vi "CSM_ExampleBrowser.vi"() -> ()   [LabVIEW 2017, in "CSM_ExampleBrowser.lvlib"]
uses:
  CSM_ExampleBrowser.lvlib
  controls/BMark_UI Data.ctl
  <vilib>/addons/analyzer/_analyzerctrls.llb/VIAnCtl Analysis App Info.ctl
  controls/BMark_Bookmark Data.ctl
  controls/BMark_VI_Identifier.ctl
  <vilib>/Utility/miscctls.llb/LVPoint32TypeDef.ctl
  _csmDoc/_Typedef/DocElement.ctl
  <vilib>/Utility/miscctls.llb/LVRowAndColumnUnsignedTypeDef.ctl
  globals/User Visible Strings.vi
  _Shared/CSM Shared.lvlib
  Communicable State Machine.lvlib
  _ui/csm-ui-support.lvlib
  _csmDoc/csmdoc.lvlib
  c14f8e0f-ff4e-477b-a84e-2a16e0658fda.vi
  _file/csm-file-support.lvlib
panel:
  in  "Localization Tool":bool
  in  "Refresh Button":bool
  in  "Zoom Factor":dbl(slide)=0.5 min=0.5 max=1.2 step=0.01 scale=0.5..1.2
  in  "ExampleTree":string(tree)
  in  "BookmarkList":i32(listbox)
  out "Preview":picture
  out "Doc":string
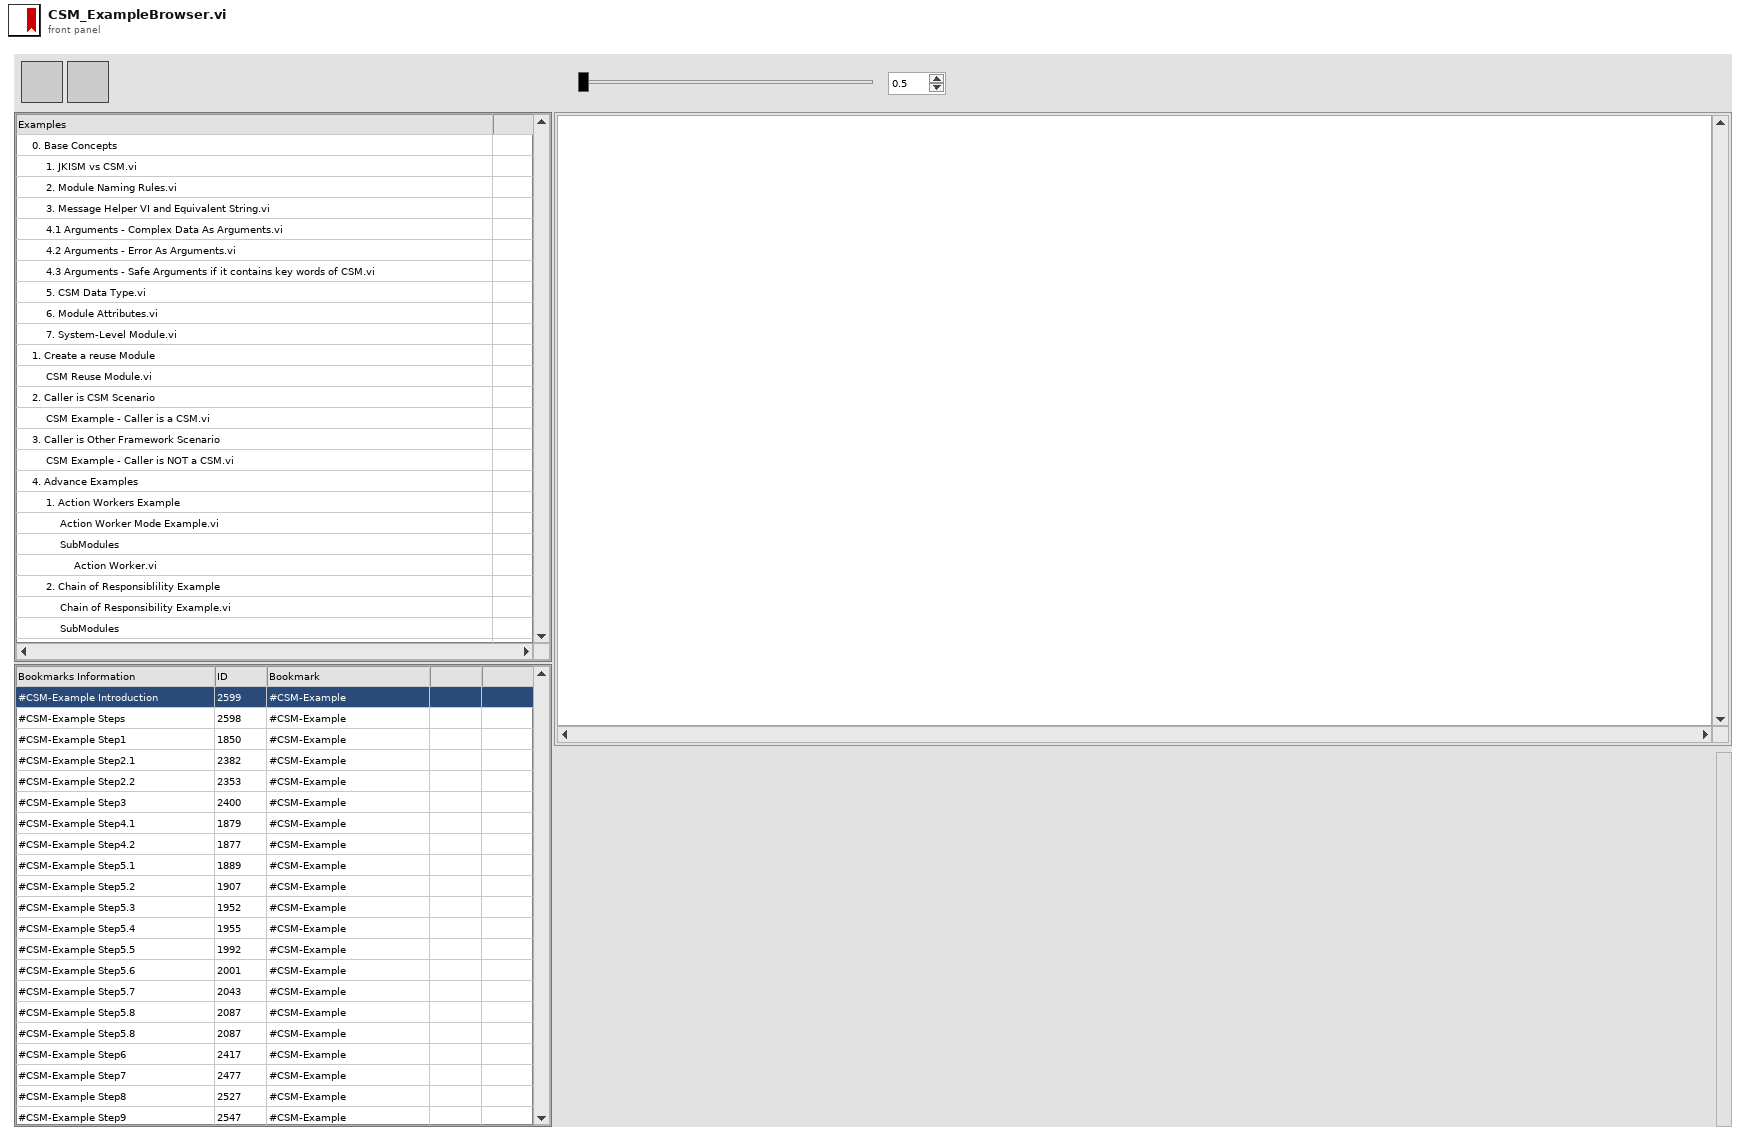
[diagram p1: front panel]
types:
  T1 = typedef "CSM_ExampleBrowser.lvlib/BMark_UI Data.ctl" = cluster{"More information":refnum<vi>, "Front Panel":refnum<vi>, "all projects":T2[], "bookmarks":T3[], "App Info":T2, "Preview image":refnum<vi>}
  T2 = typedef "VIAnCtl Analysis App Info.ctl" = cluster{"Project Name":string, "Target Name":string}
  T3 = typedef "CSM_ExampleBrowser.lvlib/BMark_Bookmark Data.ctl" = cluster{"bookmark tag":string, "full text":string, "bookmark ref":i32, "VI display name":string, "VI identifier":T4}
  T4 = typedef "CSM_ExampleBrowser.lvlib/BMark_VI_Identifier.ctl" = cluster{"Name":string, "Path":path, "App Info":T2}
  T5 = enum32{"Invalid", "Default", "Floating", "Floating/Auto-Hide", "Modal"}
  T6 = enum32{"Invalid", "Standard", "Closed", "Hidden", "Minimized", "Maximized"}
  T7 = enum32{"invalid app kind", "Development System", "Run Time System", "Student Edition", "Embedded LabVIEW", "Evaluation", "Custom"}
  T8 = enum8{"Enabled", "Disabled", "Disabled and Grayed Out"}
  T9 = typedef "csmdoc.lvlib/DocElement.ctl" = cluster{"ID":string, "Content":string[], "SubIDs":string[], "Path":string[]}
  T10 = typedef "LVRowAndColumnUnsignedTypeDef.ctl" = cluster{"Row":u32, "Column":u32}
  T11 = typedef "LVPoint32TypeDef.ctl" = cluster{"Horizontal":i32, "Vertical":i32}
  T12 = typedef "LVPointTypeDef.ctl" = cluster{"Horizontal":i16, "Vertical":i16}
  T13 = cluster{"Core":cluster{"Current VI Reference":refnum<vi>, "Close Panel on Exit?":bool}, "root":path, "ExampleMarkdowns":path[], "PreviewMouseDown":bool, "PreviewMouseDownCoords":T11, "PreviewMouseDownOrigin":T11, "DocMap":variant, "tempfile":path}
  T14 = typedef "LVRectTypeDef.ctl" = cluster{"Left":i16, "Top":i16, "Right":i16, "Bottom":i16}
  T15 = cluster{"Current VI Reference":refnum<vi>, "Close Panel on Exit?":bool}
  T16 = cluster{"Core":cluster{"Current VI Reference":refnum<vi>, "Close Panel on Exit?":bool}, "root":path, "PreviewMouseDown":bool, "PreviewMouseDownCoords":T11, "PreviewMouseDownOrigin":T11}
  T17 = typedef "csmdoc.lvlib/DocNote.ctl" = cluster{"ID":string, "Content":string, "Type":string}
  T18 = typedef "LVBookmarkInfoTypeDef.ctl" = cluster{"Bookmark Reference":u32, "Bookmark Tag":string, "Label Text":string}[]
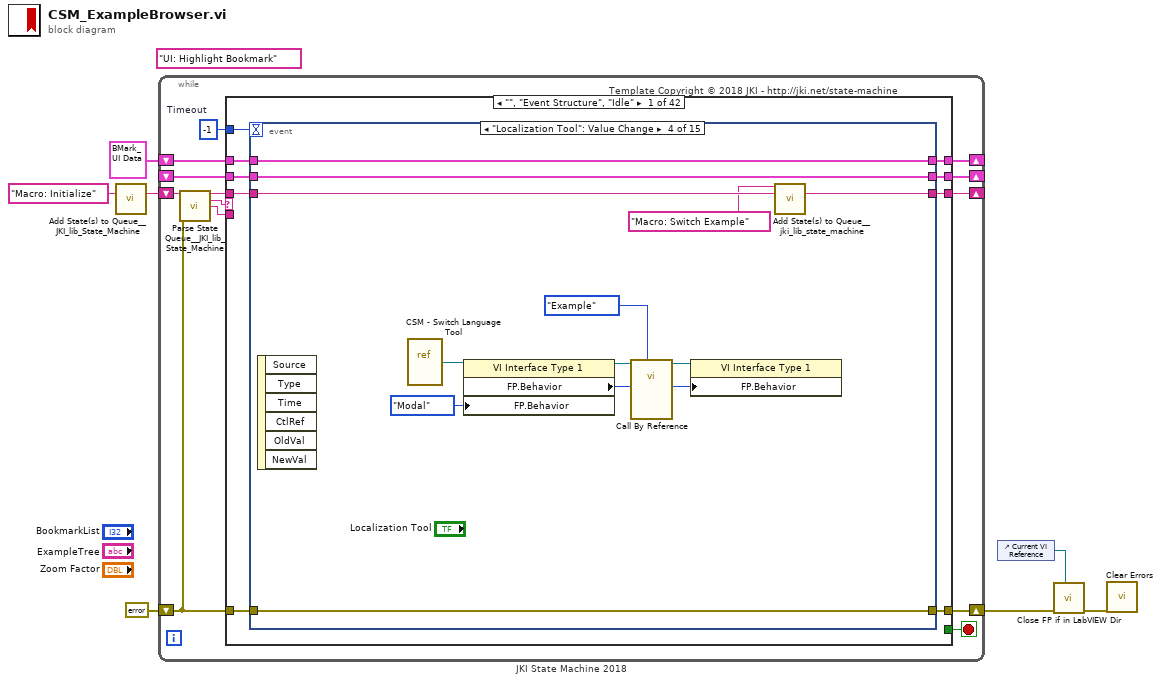
[diagram p0: block diagram]
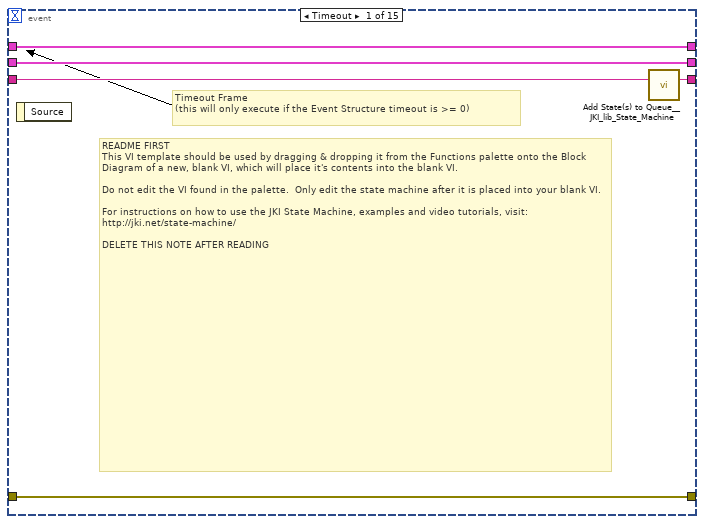
[diagram p2: hidden frame]
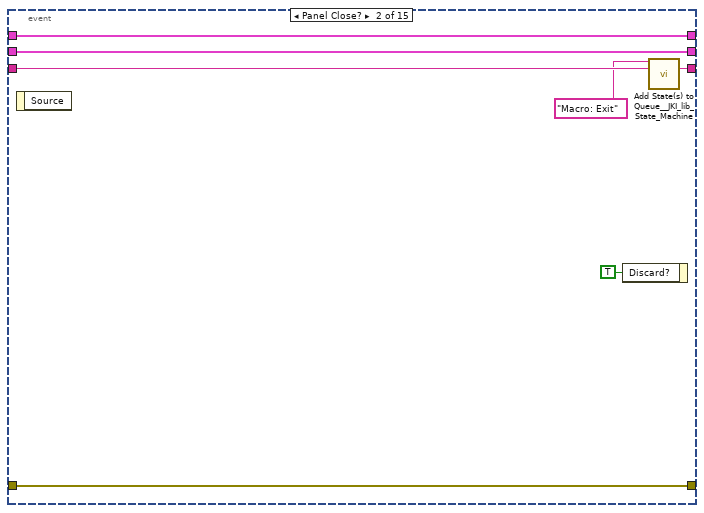
[diagram p3: hidden frame]
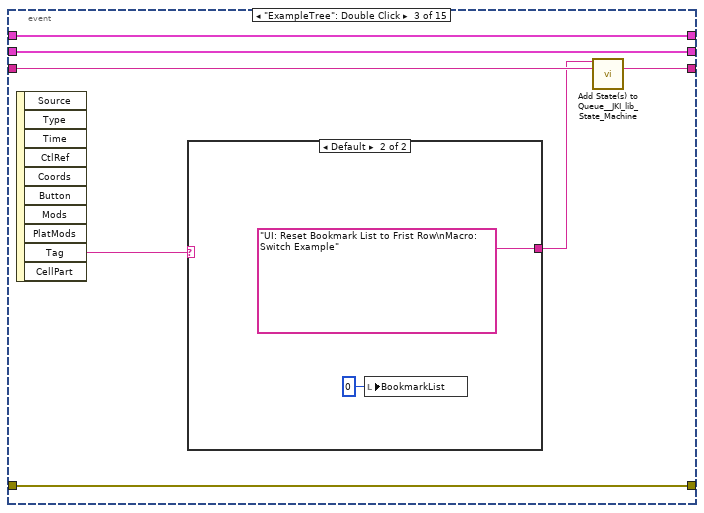
[diagram p4: hidden frame]
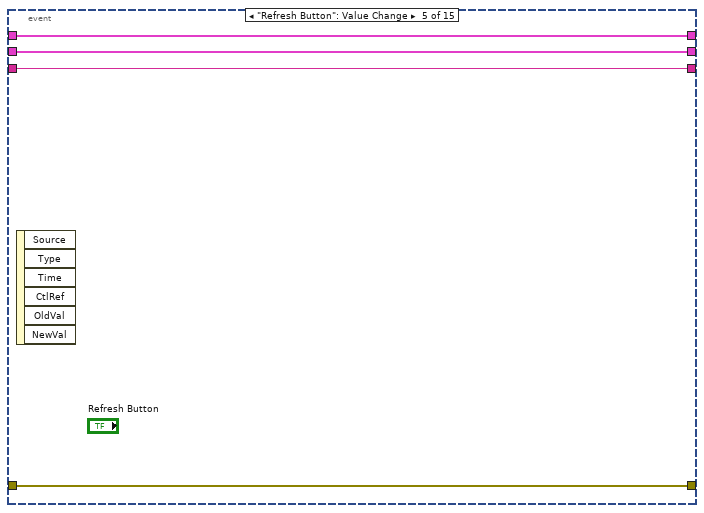
[diagram p6: hidden frame]
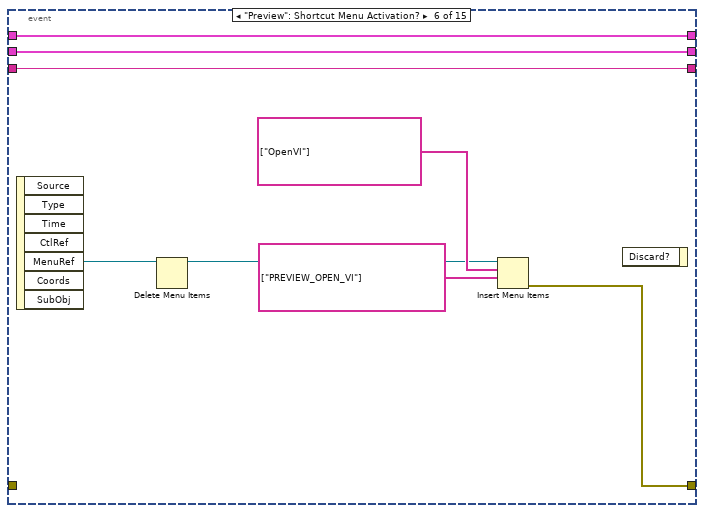
[diagram p7: hidden frame]
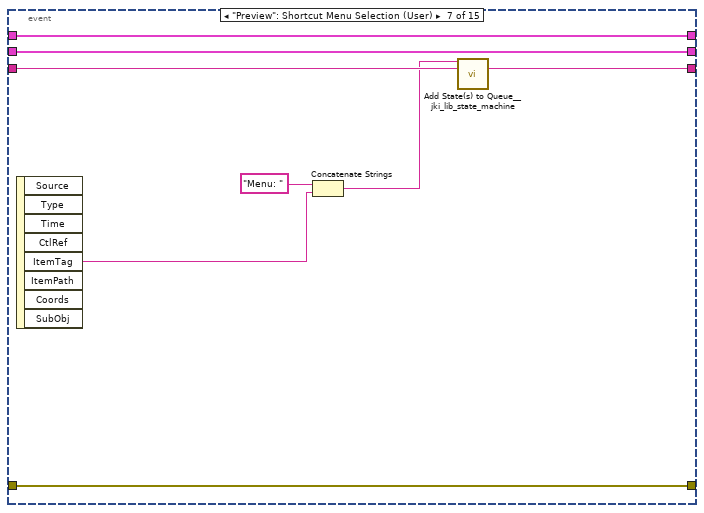
[diagram p8: hidden frame]
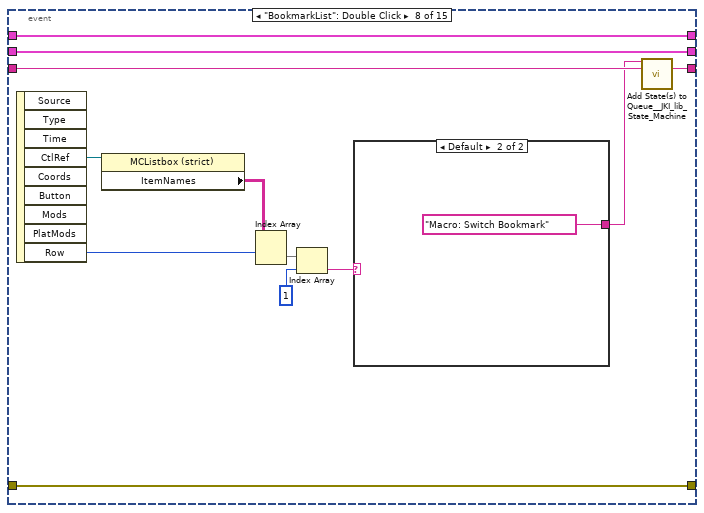
[diagram p9: hidden frame]
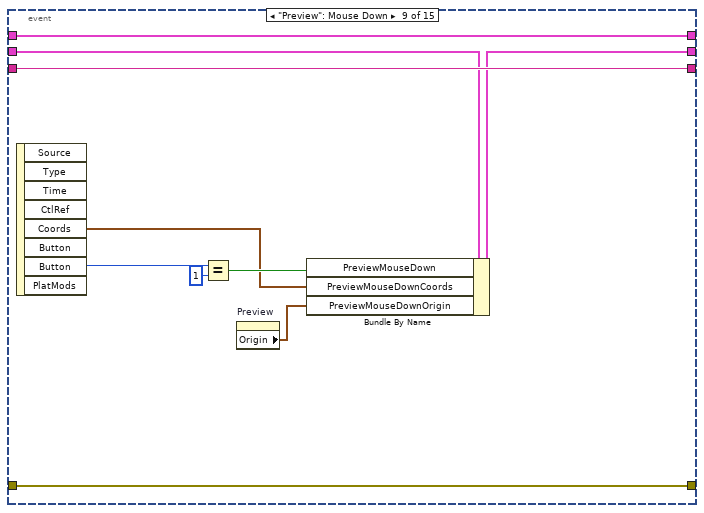
[diagram p11: hidden frame]
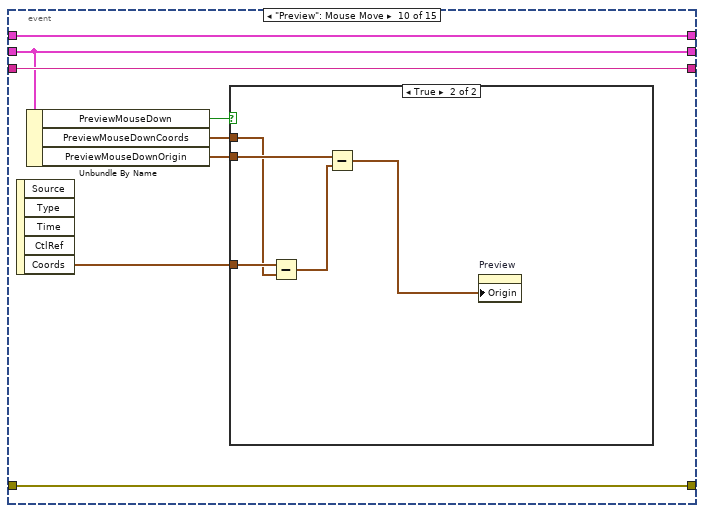
[diagram p12: hidden frame]
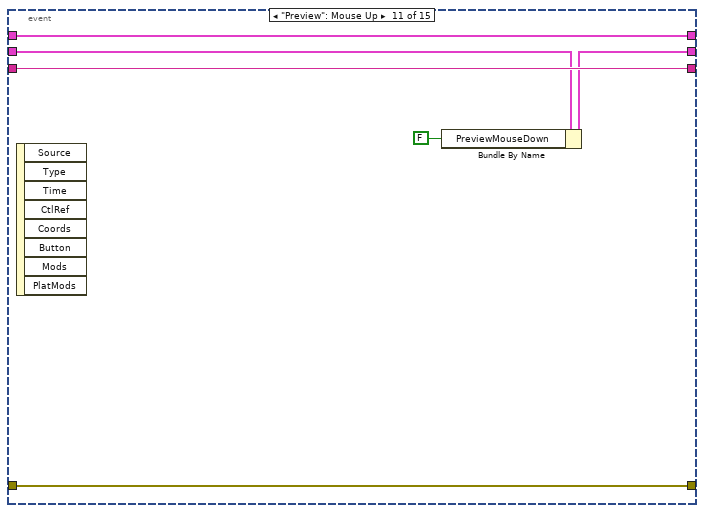
[diagram p14: hidden frame]
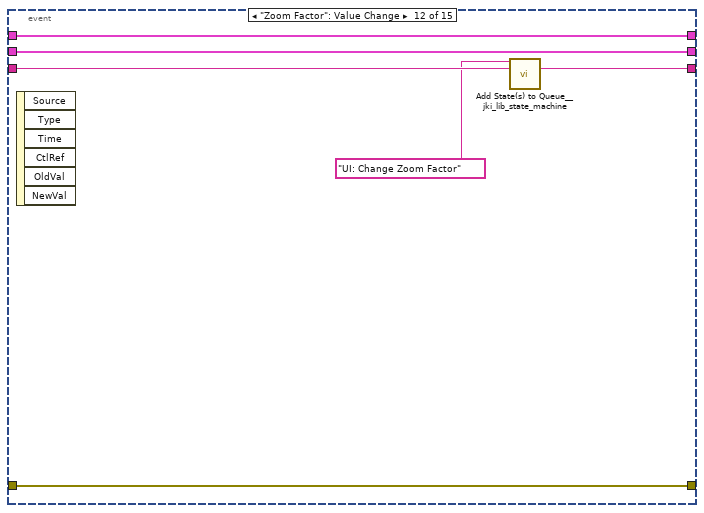
[diagram p15: hidden frame]
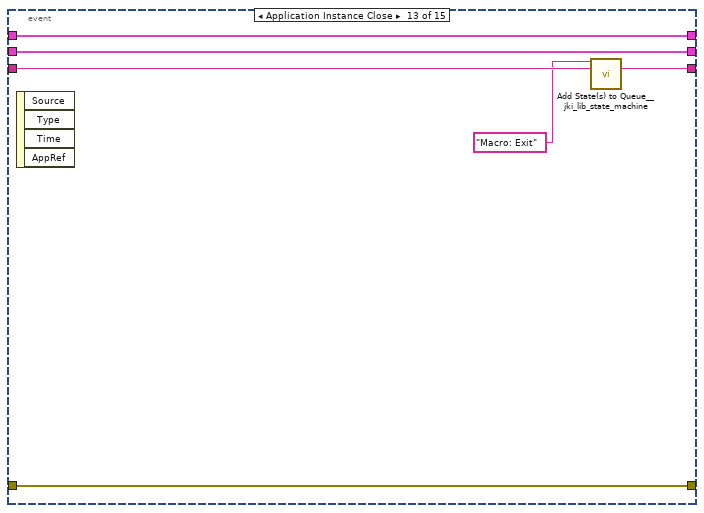
[diagram p16: hidden frame]
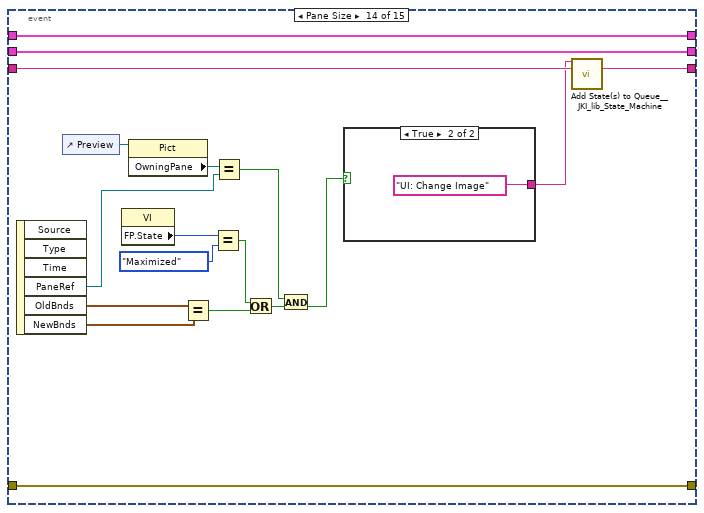
[diagram p17: hidden frame]
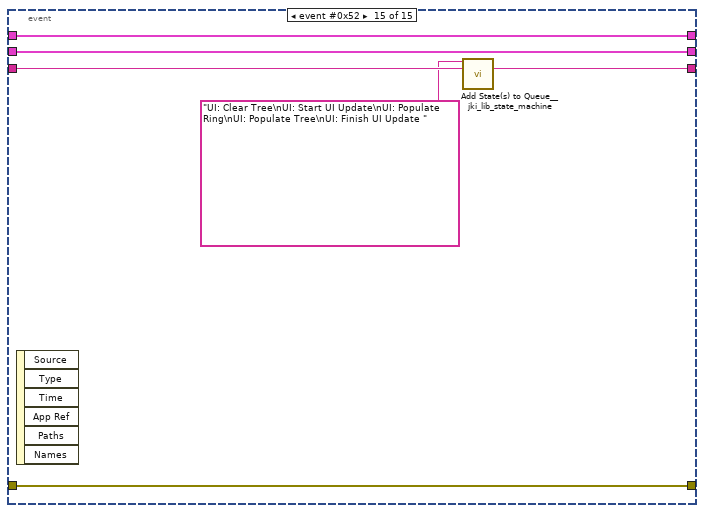
[diagram p19: hidden frame]
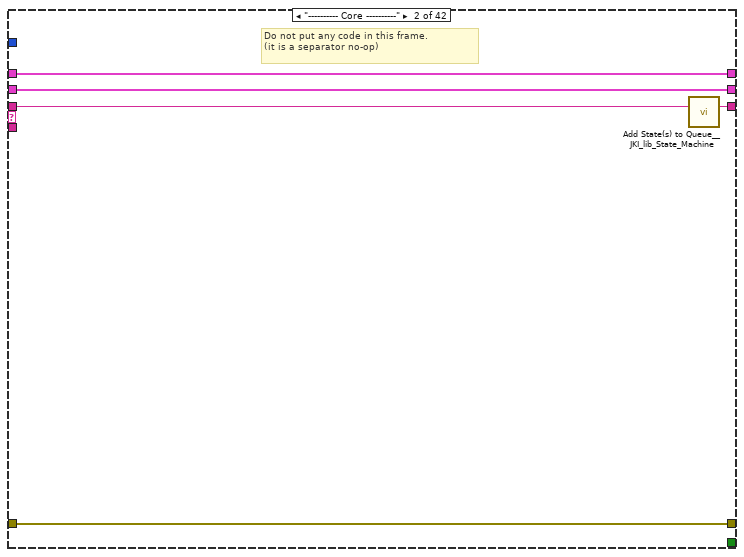
[diagram p20: hidden frame]
diagram:
  (unwired) "UI: Highlight Bookmark" ("Message")
  n1 = call <vilib>:"Add State(s) to Queue__JKI_lib_State_Machine.vi"("State(s) in (\"\")"="Macro: Initialize") -> ("States Out"=w6:string)  [unwired: 14 in]
  n2 = while "JKI State Machine 2018" {
    shift-right: [w13] -> _
    shift-left: _ -> [w12]
    shift-right: [w16] -> w1
    shift-left: errorcluster {"status"=FALSE, "code"=0, "source"=""} ("error out") -> [w10]
    shift-right: [w15] -> _
    shift-left: w6 -> [w17]
    shift-right: [w9] -> _
    shift-left: T1 {"More information"=refnum, "Front Panel"=refnum, "all projects"=[], "bookmarks"=[], "App Info"={"Project Name"="", "Target Name"=""}, "Preview image"=refnum} ("Data Cluster") -> [w8]
    stop <- w14 stop-if-true
    w11 = -1  # Timeout
    # "Template Copyright © 2018 JKI - http://jki.net/state-machine"
    n3 = call <vilib>:"Parse State Queue__JKI_lib_State_Machine.vi"("State Queue"=w17, "Error In (no error)"=w10) -> ("Remaining States"=w19:string, "Current State"=w20:string, "Arguments"=w18:string)  [unwired: 11 in]
    n4 = case shown="\"\", \"Event Structure\", \"Idle\"" w20 {
      selector: w20 -> [_ _ w168 _ _ _ _ _ _ _ _ _ _ _ _ _ _ _ _ _ _ _ _ _ _ _ _ _ _ _ _ _ _ _ _ _ _ _ _ _ _ _]
      tunnel: w19 -> [w29 w166 w172 w192 w199 w205 w210 w227 w244 w260 w274 w285 w290 w300 w302 w317 w320 w329 w338 w341 w354 w360 w376 w425 w432 w434 w452 w477 w489 w560 w568 w571 w584 w590 w596 w602 w613 w618 w626 w631 w662 w681]
      tunnel: w18 -> [_ _ _ _ _ _ _ _ _ _ _ _ _ _ _ _ _ _ _ _ _ _ w363 _ w430 _ _ w472 w483 w556 _ _ _ _ _ _ _ _ _ _ _ _]
      tunnel: w12 -> [w27 w163 w170 w185 w196 w203 w207 w211 _ w259 w272 w280 w287 w298 w306 w316 w323 w328 w337 w340 w346 w359 w375 w424 w431 w437 w448 w475 w485 w559 w567 w575 w581 w587 w593 w599 w610 w615 w620 w629 w657 w675]
      tunnel: [w26 w164 w174 w189 errorcluster {"status"=FALSE, "code"=0, "source"=""} ("error out") w202 w208 w224 w241 w261 w275 w281 w288 w297 w305 w318 w324 w330 w336 _ w345 w361 w366 _ _ _ _ w473 w486 w561 w569 w579 w582 w588 w594 w600 w611 w616 w627 _ w653 w679] -> w16
      tunnel: w10 -> [w25 w164 w173 w189 w195 w202 w208 w224 w241 w261 w275 w282 w288 w297 _ w318 w324 w330 _ _ _ w361 _ _ _ _ _ w474 w487 w561 w569 w579 w582 w588 w594 w600 w611 w616 w627 _ _ w679]
      tunnel: [w28 w165 w171 w191 w198 w204 w209 w226 w243 w260 w274 w284 w289 w299 w303 w317 w321 w329 w338 w341 w354 w360 w376 w425 w432 w435 w452 w476 w488 w560 w568 w572 w583 w589 w595 w601 w612 w617 w626 w631 w661 w680] -> w15
      tunnel: [_ _ _ _ _ TRUE _ _ _ _ _ _ _ _ _ _ _ _ _ _ _ _ _ _ _ _ _ _ _ _ _ _ _ _ _ _ _ _ _ _ _ _] -> w14
      tunnel: [w24 w163 w170 w190 w196 w203 w207 w211 w237 w257 w269 w280 w287 w298 w306 w316 w323 w328 w337 w340 w346 w359 w375 w424 w431 w437 w450 w475 w485 w559 w567 w575 w581 w587 w593 w599 w610 w615 w620 w628 w655 w675] -> w13
      tunnel: w11 -> [w23 _ _ _ _ _ _ _ _ _ _ _ _ _ _ _ _ _ _ _ _ _ _ _ _ _ _ _ _ _ _ _ _ _ _ _ _ _ _ _ _ _]
      tunnel: [w22 w162 w167 w179 w193 w200 w206 w215 w231 w258 w273 w279 w286 w296 w304 w308 w322 w325 w333 w339 w348 w356 w367 w423 w429 w447 w451 w471 w482 w558 w566 w578 w580 w585 w591 w597 w603 w614 w625 w630 w660 w678] -> w9
      tunnel: w8 -> [w21 w162 w167 w179 w193 w200 w206 w216 w231 w258 w273 w279 w286 w296 w304 w308 w322 w325 w332 w339 w348 w356 w367 w423 w429 w447 w451 w471 w482 w558 w566 w578 w580 w585 w591 w597 w603 w614 w625 w630 w660 w678]
      frame "", "Event Structure", "Idle" {
        n5 = event shown="[3] \"Localization Tool\": Value Change" {
          selector: _ -> [_ _ _ _ _ _ _ _ _ _ _ _ _ _ _]
          dyn-events: _ -> [_ _ _ _ _ _ _ _ _ _ _ _ _ _ _]
          timeout: w23 -> [_ _ _ _ _ _ _ _ _ _ _ _ _ _ _]
          tunnel: w29 -> [w34 w41 w44 w52 w66 w74 w78 w90 w105 w113 w124 w126 w132 w144 w157]
          tunnel: [w33 w40 w45 w53 w66 w74 w79 w91 w105 w113 w124 w127 w133 w145 w158] -> w28
          tunnel: w27 -> [w31 w38 w47 w61 w64 w73 w81 w93 w103 w110 w122 w129 w135 w153 w160]
          tunnel: [w32 w39 w48 w62 w65 w68 w82 w94 w104 w112 w123 w130 w136 w154 w161] -> w26
          tunnel: w25 -> [w32 w39 w48 w62 w65 _ w82 w94 w104 w112 w123 w130 w136 w154 w161]
          tunnel: [w31 w38 w47 w61 w64 w73 w81 w93 w101 w110 w120 w129 w135 w153 w160] -> w24
          tunnel: [w30 w35 w46 w60 w63 w72 w80 w92 w102 w111 w121 w128 w134 w152 w159] -> w22
          tunnel: w21 -> [w30 w35 w46 w60 w63 w72 w80 w92 w102 w111 w121 w128 w134 w152 w159]
          event Timeout {
            # "README FIRST\nThis VI template should be used by dragging & dropping it from the Functions palette onto the Block Diagram of a new, blank VI, which will place it's contents into the blank VI.\n\nDo not edit the VI found in the palette.  Only edit the state machine after it is placed into your blank VI.\n\nFor instructions on how to use the JKI State Machine, examples and video tutorials, visit:\nhttp://jki.net/state-machine/\n\nDELETE THIS NOTE AFTER READING"
            # "Timeout Frame\n(this will only execute if the Event Structure timeout is >= 0)"
            n6 = event-data() -> ()  [unwired: 1 in, 1 out]
            n7 = call <vilib>:"Add State(s) to Queue__JKI_lib_State_Machine.vi"("State(s) in (\"\")"=w34) -> ("States Out"=w33:string)  [unwired: 14 in]
          }
          event Panel Close? {
            n8 = event-data() -> ()  [unwired: 1 in, 1 out]
            n9 = event-data("Discard?"=TRUE) -> ()  [unwired: 1 in, 1 out]
            n10 = call <vilib>:"Add State(s) to Queue__JKI_lib_State_Machine.vi"("State(s) in Front (\"\")"="Macro: Exit", "State(s) in (\"\")"=w41) -> ("States Out"=w40:string)  [unwired: 13 in]
          }
          event "ExampleTree": Double Click {
            n11 = event-data() -> ("Tag"=w42:string)  [unwired: 1 in, 9 out]
            n12 = case shown="Default" w42 {
              tunnel: [_ "UI: Reset Bookmark List to Frist Row\nMacro: Switch Example" ("Message")] -> w43
              frame "" {
              }
              frame Default {
                n13 = local write "BookmarkList"(0 ("BookmarkList")) -> ()
              }
            }
            n14 = call <vilib>:"Add State(s) to Queue__JKI_lib_State_Machine.vi"("State(s) in Front (\"\")"=w43, "State(s) in (\"\")"=w44) -> ("States Out"=w45:string)  [unwired: 13 in]
          }
          event "Localization Tool": Value Change {
            n15 = event-data() -> ()  [unwired: 1 in, 6 out]
            n16 = vi-ref "CSM - Switch Language Tool.vi"() -> (w59:refnum<vi>)
            n17 = property class="VI Interface Type 1"(reference=w59, "FP.Behavior"=T5."Modal" ("Front Panel Window:Behavior")) -> (reference out=w56:refnum<vi>, "FP.Behavior"=w57:T5)  [unwired: 1 in, 1 out]
            n18 = call-by-ref "?"(reference=w56, "Type"=enum16{"VI Description", "Example"}."Example") -> (reference out=w55:refnum<vi>)  [unwired: 12 in, 1 out]
            n19 = property class="VI Interface Type 1"(reference=w55, "FP.Behavior"=w57) -> ()  [unwired: 1 in, 2 out]
            n20 = call <vilib>:"Add State(s) to Queue__jki_lib_state_machine.vi"("State(s) in Front (\"\")"="Macro: Switch Example" ("State(s) in Front (\"\")"), "State(s) in (\"\")"=w52) -> ("States Out"=w53:string)  [unwired: 13 in]
          }
          event "Refresh Button": Value Change {
            n21 = event-data() -> ()  [unwired: 1 in, 6 out]
          }
          event "Preview": Shortcut Menu Activation? {
            n22 = event-data() -> ("MenuRef"=w71:refnum<k9>)  [unwired: 1 in, 6 out]
            n23 = Delete Menu Items(9:w71) -> (3:w67:refnum<k9>)  [unwired: 3 in, 1 out]
            n24 = Insert Menu Items(7:string[] ["PREVIEW_OPEN_VI"] ("item names"), 8:string[] ["OpenVI"] ("item names"), 9:w67) -> (0:w68:errorcluster)  [unwired: 3 in, 2 out]
            n25 = event-data() -> ()  [unwired: 2 in, 1 out]
          }
          event "Preview": Shortcut Menu Selection (User) {
            n26 = event-data() -> ("ItemTag"=w76:string)  [unwired: 1 in, 7 out]
            n27 = Concatenate Strings("Menu: ", w76) -> (w75:string)
            n28 = call <vilib>:"Add State(s) to Queue__jki_lib_state_machine.vi"("State(s) in Front (\"\")"=w75, "State(s) in (\"\")"=w78) -> ("States Out"=w79:string)  [unwired: 13 in]
          }
          event "BookmarkList": Double Click {
            n29 = event-data() -> ("CtlRef"=w88:refnum<vi>, "Row"=w86:i32)  [unwired: 1 in, 7 out]
            n30 = property class="MCListbox (strict)"(reference=w88) -> ("ItemNames"=w87:string[][])  [unwired: 1 in, 2 out]
            n31 = Index Array(array=w87, index (row)=w86) -> (element=w85:string[])  [unwired: 1 in]
            n32 = Index Array(array=w85, index=1) -> (element=w84:string)
            n33 = case shown="Default" w84 {
              tunnel: [_ "Macro: Switch Bookmark" ("Message")] -> w89
              frame "" {
              }
              frame Default {
              }
            }
            n34 = call <vilib>:"Add State(s) to Queue__JKI_lib_State_Machine.vi"("State(s) in Front (\"\")"=w89, "State(s) in (\"\")"=w90) -> ("States Out"=w91:string)  [unwired: 13 in]
          }
          event "Preview": Mouse Down {
            n35 = event-data() -> ("Coords"=w97:T11, "Button"=w100:u16)  [unwired: 1 in, 6 out]
            n36 = Equal?(x=w100, y=u16 1) -> (x = y?=w99:bool)
            n37 = property on="Preview" class="Pict"() -> ("Origin"=w96:T12)  [unwired: 2 in, 2 out]
            n38 = Bundle By Name(cluster=w103, "PreviewMouseDown"=w99, "PreviewMouseDownCoords"=w97, "PreviewMouseDownOrigin"=w96) -> (w101:T13)
          }
          event "Preview": Mouse Move {
            n39 = event-data() -> ("Coords"=w107:T11)  [unwired: 1 in, 4 out]
            n40 = Unbundle By Name(w110) -> ("PreviewMouseDown"=w109:bool, "PreviewMouseDownCoords"=w108:T11, "PreviewMouseDownOrigin"=w106:T11)
            n41 = case shown="True" w109 {
              tunnel: w108 -> [_ w116]
              tunnel: w107 -> [_ w117]
              tunnel: w106 -> [_ w118]
              frame False {
              }
              frame True {
                n42 = Subtract(x=w117, y=w116) -> (x-y=w115:T11)
                n43 = Subtract(x=w118, y=w115) -> (x-y=w114:T11)
                n44 = property on="Preview" class="Pict"("Origin"=w114) -> ()  [unwired: 2 in, 2 out]
              }
            }
          }
          event "Preview": Mouse Up {
            n45 = event-data() -> ()  [unwired: 1 in, 8 out]
            n46 = Bundle By Name(cluster=w122, "PreviewMouseDown"=FALSE) -> (w120:T13)
          }
          event "Zoom Factor": Value Change {
            n47 = event-data() -> ()  [unwired: 1 in, 6 out]
            n48 = call <vilib>:"Add State(s) to Queue__jki_lib_state_machine.vi"("State(s) in Front (\"\")"="UI: Change Zoom Factor" ("State(s) in Front (\"\")"), "State(s) in (\"\")"=w126) -> ("States Out"=w127:string)  [unwired: 13 in]
          }
          event Application Instance Close {
            n49 = event-data() -> ()  [unwired: 1 in, 4 out]
            n50 = call <vilib>:"Add State(s) to Queue__jki_lib_state_machine.vi"("State(s) in Front (\"\")"="Macro: Exit" ("State(s) in Front (\"\")"), "State(s) in (\"\")"=w132) -> ("States Out"=w133:string)  [unwired: 13 in]
          }
          event Pane Size {
            n51 = event-data() -> ("PaneRef"=w139:refnum<vi>, "OldBnds"=w147:T14, "NewBnds"=w146:T14)  [unwired: 1 in, 3 out]
            n52 = control-ref of="Preview"() -> (w141:refnum<vi>)
            n53 = property class="VI"() -> ("FP.State"=w151:T6)  [unwired: 2 in, 2 out]
            n54 = property class="Pict"(reference=w141) -> ("OwningPane"=w140:refnum<vi>)  [unwired: 1 in, 2 out]
            n55 = Equal?(x=w147, y=w146) -> (x = y?=w148:bool)
            n56 = Equal?(x=w151, y=T6."Maximized" ("Front Panel Window:State")) -> (x = y?=w149:bool)
            n57 = Equal?(x=w140, y=w139) -> (x = y?=w137:bool)
            n58 = Or(x=w149, y=w148) -> (x .or. y?=w142:bool)
            n59 = And(x=w137, y=w142) -> (x .and. y?=w138:bool)
            n60 = case shown="True" w138 {
              tunnel: [_ "UI: Change Image" ("Message")] -> w143
              frame False {
              }
              frame True {
              }
            }
            n61 = call <vilib>:"Add State(s) to Queue__JKI_lib_State_Machine.vi"("State(s) in Front (\"\")"=w143, "State(s) in (\"\")"=w144) -> ("States Out"=w145:string)  [unwired: 13 in]
          }
          event event #0x52 {
            n62 = event-data() -> ()  [unwired: 1 in, 6 out]
            n63 = call <vilib>:"Add State(s) to Queue__jki_lib_state_machine.vi"("State(s) in Front (\"\")"="UI: Clear Tree\nUI: Start UI Update\nUI: Populate Ring\nUI: Populate Tree\nUI: Finish UI Update " ("State(s) in Front (\"\")"), "State(s) in (\"\")"=w157) -> ("States Out"=w158:string)  [unwired: 13 in]
          }
        }
      }
      frame "---------- Core ----------" {
        # "Do not put any code in this frame.\n(it is a separator no-op)"
        n64 = call <vilib>:"Add State(s) to Queue__JKI_lib_State_Machine.vi"("State(s) in (\"\")"=w166) -> ("States Out"=w165:string)  [unwired: 14 in]
      }
      frame Default {
        w177 = 42 items=["No error", "Argument error", "Memory is full", "Out of zone", "End of file", "File already open", "Generic file I/O error", "File not found", "File permission error", "Disk is full", "Duplicate path", "Too many files open", "System feature not enabled", "Resource file not found", "Cannot add resource", "Resource not found", "Image not found", "Image memory error", "Pen does not exist", "Config type invalid", "Config token not found", "Config parse error", "Config memory error", "Bad external code format", "Bad external code offset", "External code not present", "Null window", "Destroy window error", "Null menu", "Print aborted", "Bad print record", "Print driver error", "Windows error during printing", "Memory error during printing", "Print dialog error", "Generic print error", "Invalid device refnum", "Device not found", "Device parameter error", "Device unit error", "Cannot open device", "Device call aborted", "Generic error", "Cancelled by user", "Object ID too low", "Object ID too high", "Object not in heap", "Unknown heap", "Unknown object (invalid DefProc)", "Unknown object (DefProc not in table)", "Message out of range", "Invalid (null) method", "Unknown message", "Manager call not supported", "Bad address", "Network operation in progress", "Network operation timed out", "Connection is busy", "Network attribute not supported", "Network error", "Address in use", "System out of memory", "Connection aborted", "Connection refused", "Not connected", "Already connected", "Connection closed", "Initialization error (interapplication manager)", "Bad occurrence", "Wait on unbound occurrence handler", "Occurrence queue overflow", "Datalog type conflict", "Unused", "Unrecognized type (interapplication manager)", "Memory corrupt", "Failed to make temporary DLL", "Old CIN version", "Drag socket not found", "Failed to load drop-object", "Failed to register OLE object", "Failed to release OLE object", "Format specifier type mismatch", "Unknown format specifier", "Too few format specifiers", "Too many format specifiers", "Scan failed", "Newer CIN version", "Error converting to variant", "Runtime menu error", "Password tampered", "Variant attribute not found", "Incompatible variant data type", "Event data is not available", "Event Store is not present", "Occurrence is not found", "Event Queue is not created", "Event info is not available", "Refnum passed is NULL", "Error retrieving Class GUID", "Error retrieving CoClass GUID", "Error retrieving TypeLib GUID.", "Bad built application magic bytes.", "Specific driver is different from the specific driver associated with the Logical Name.", "There is no session opened to the class driver.", "Max Error", "MAX - Error with config objects", "MAX - Error loading configuration", "MAX - Group not supported"]
        # "Current State"
        # "Do not delete, rename, or modify this frame.\n(this is used to capture unhandled states and typos)"
        # "Handle mistyped state name (developer tool)"
        n65 = Format Into String(format string="Software Exception: Unhandled State \"%s\"." ("message"), error in=w173, w168) -> (resulting string=w176:string, error out=w175:errorcluster)  [unwired: 1 in]
        n66 = call <vilib>:"Error Cluster From Error Code.vi"("show call chain? (False)"=TRUE, "error in (no error)"=w175, "error message (\"\")"=w176, "error code (0)"=w177) -> ("error out"=w174:errorcluster)  [unwired: 5 in]
        n67 = call <vilib>:"Add State(s) to Queue__JKI_lib_State_Machine.vi"("State(s) in (\"\")"=w172) -> ("States Out"=w171:string)  [unwired: 14 in]
      }
      frame "Initialize Core Data" {
        # "Do not delete, rename, or modify this frame.\n(this is used to determine panel behavior on exit)"
        # "originally closed?"
        # "exe?"
        # "If panel starts closed or is an EXE, then close it when we exit"
        n68 = property class="VI"() -> ("FP.State"=w182:T6)  [unwired: 2 in, 2 out]
        n69 = property class="App"() -> ("App.Kind"=w188:T7)  [unwired: 2 in, 2 out]
        n70 = control-ref of="Current VI Reference"() -> (w183:refnum<vi>)
        n71 = Equal?(x=w182, y=T6."Closed" ("Front Panel Window:State")) -> (x = y?=w180:bool)
        n72 = Equal?(x=w188, y=T7."Run Time System" ("Application:Kind")) -> (x = y?=w186:bool)
        n73 = Or(x=w180, y=w186) -> (x .or. y?=w184:bool)
        n74 = Bundle By Name(cluster=w185, "Core.Current VI Reference"=w183, "Core.Close Panel on Exit?"=w184) -> (w190:T13)
        n75 = call <vilib>:"Add State(s) to Queue__JKI_lib_State_Machine.vi"("State(s) in (\"\")"=w192) -> ("States Out"=w191:string)  [unwired: 14 in]
      }
      frame "Error Handler" {
        # "Unhandled Error -- Display it"
        # "Handle any errors here.\nYou can also output any states to clean-up after errors occur"
        # "Clear error"
        n76 = call <vilib>:"General Error Handler.vi"("error in (no error)"=w195) -> ()  [unwired: 10 in, 5 out]
        n77 = call <vilib>:"Add State(s) to Queue__JKI_lib_State_Machine.vi"("State(s) in Front (\"\")"="/* Post Error States", "State(s) in (\"\")"=w199) -> ("States Out"=w198:string)  [unwired: 13 in]
      }
      frame "Exit" {
        # "Do not put any code in this frame.\n(No errors that occur here will be handled.)"
        n78 = call <vilib>:"Add State(s) to Queue__JKI_lib_State_Machine.vi"("State(s) in (\"\")"=w205) -> ("States Out"=w204:string)  [unwired: 14 in]
      }
      frame "---------- Data ----------" {
        # "Do not put any code in this frame.\n(It is a separator no-op. You can make a copy of this frame to create a new Data frame)"
        n79 = call <vilib>:"Add State(s) to Queue__JKI_lib_State_Machine.vi"("State(s) in (\"\")"=w210) -> ("States Out"=w209:string)  [unwired: 14 in]
      }
      frame "Data: Initialize Refs" {
        w212 = T11 {"Horizontal"=0, "Vertical"=0}  # PreviewMouseDownOrigin
        w213 = T11 {"Horizontal"=0, "Vertical"=0}  # PreviewMouseDownCoords
        w214 = FALSE  # PreviewMouseDown
        w223 = T15 {"Current VI Reference"=refnum, "Close Panel on Exit?"=FALSE}  # Core
        w219 = path ""  # root
        # "Initialize the shift-register data, here.\n(data names are defined by what you wire into the bundle function)"
        n80 = property class="VI"() -> ("Panel"=w217:refnum<vi>)  [unwired: 2 in, 2 out]
        n81 = control-ref of="Preview"() -> (w218:refnum<vi>)
        n82 = Bundle By Name(cluster=w216, "Front Panel"=w217, "Preview image"=w218) -> (w215:T1)
        n83 = Bundle("Core"=w223, "root"=w219, "PreviewMouseDown"=w214, "PreviewMouseDownCoords"=w213, "PreviewMouseDownOrigin"=w212) -> (w225:T16)  [unwired: 1 in]
        n84 = call "CSM - user.lib Dir.vi"() -> ("<LabVIEW>"=w222:path)  [unwired: 2 in, 1 out]
        n85 = Build Path(base path=w222, name or relative path="Example") -> (appended path=w220:path)
        n86 = Bundle By Name(cluster=w225, "root"=w220) -> ()  [unwired: 1 out]
        n87 = call <vilib>:"Add State(s) to Queue__JKI_lib_State_Machine.vi"("State(s) in (\"\")"=w227) -> ("States Out"=w226:string)  [unwired: 14 in]
      }
      frame "Data: Initialize" {
        w228 = path ""  # tempfile
        w229 = variant  # DocMap
        w230 = path[] []  # ExampleMarkdowns
        w232 = T11 {"Horizontal"=0, "Vertical"=0}  # PreviewMouseDownOrigin
        w233 = T11 {"Horizontal"=0, "Vertical"=0}  # PreviewMouseDownCoords
        w234 = FALSE  # PreviewMouseDown
        w240 = T15 {"Current VI Reference"=refnum, "Close Panel on Exit?"=FALSE}  # Core
        w235 = path ""  # root
        n88 = Bundle("Core"=w240, "root"=w235, "ExampleMarkdowns"=w230, "PreviewMouseDown"=w234, "PreviewMouseDownCoords"=w233, "PreviewMouseDownOrigin"=w232, "DocMap"=w229, "tempfile"=w228) -> (w242:T13)  [unwired: 1 in]
        n89 = call "CSM - user.lib Dir.vi"() -> ("<LabVIEW>"=w239:path)  [unwired: 2 in, 1 out]
        n90 = Build Path(base path=w239, name or relative path="examples\\NEVSTOP\\Communicable State Machine(CSM)") -> (appended path=w236:path)
        n91 = Bundle By Name(cluster=w242, "root"=w236) -> (w237:T13)
        n92 = call <vilib>:"Add State(s) to Queue__JKI_lib_State_Machine.vi"("State(s) in (\"\")"=w244) -> ("States Out"=w243:string)  [unwired: 14 in]
      }
      frame "Data: Search Example Markdowns" {
        w250 = cluster{"left":string, "right":string} {"left"="(", "right"=")"} ("Cluster")
        n93 = call "CSM - user.lib Dir.vi"() -> ("<LabVIEW>"=w256:path)  [unwired: 2 in, 1 out]
        n94 = Build Path(base path=w256, name or relative path="help\\NEVSTOP\\Communicable State Machine(CSM)\\Examples") -> (appended path=w254:path)
        n95 = call "_Match String Inside Pattern.vi"("Cluster"=w250, "string"="") -> ("String inside"=w249:string)  [unwired: 8 in, 1 out]
        n96 = Unbundle(w250) -> ("left"=w247:string, "right"=w248:string)
        n97 = call <vilib>:"Recursive File List.vi"("pattern"="*.md", "Folder Path"=w254) -> ("All Files in Dir"=w252:path[])  [unwired: 5 in, 4 out]
        n98 = Concatenate Strings(w247, w249, w248) -> (w246:string)
        n99 = for {
          tunnel: w252 -> [w266] mode=indexing
          tunnel: [w266] -> w251 mode=indexing if=w262
          tunnel: w246 -> [w264]
          n100 = Strip Path(path=w266) -> (name=w265:string)  [unwired: 1 out]
          n101 = Match Pattern(string=w265, regular expression=w264) -> (offset past match=w263:i32)  [unwired: 1 in, 3 out]
          n102 = Greater Or Equal To 0?(x=w263) -> (x >= 0?=w262:bool)
        }
        n103 = Bundle By Name(cluster=w259, "ExampleMarkdowns"=w251) -> (w257:T13)
      }
      frame "Data: Load Example Markdown Files" {
        n104 = Unbundle By Name(w272) -> ("ExampleMarkdowns"=w271:path[])
        n105 = for {
          tunnel: w271 -> [w278] mode=indexing
          tunnel: [w277] -> w270 mode=concatenating
          tunnel: [w276] -> w267 mode=concatenating
          n106 = call "_Load Markdown File.vi"("Path"=w278) -> ("Array 2"=w276:T17[], "Array"=w277:T9[])  [unwired: 8 in, 1 out]
        }
        n107 = call "_Generate DocMap.vi"("Array 2"=w267, "Array"=w270) -> ("Variant"=w268:variant)  [unwired: 9 in]
        n108 = Bundle By Name(cluster=w272, "DocMap"=w268) -> (w269:T13)
      }
      frame "Data: Cleanup" {
        # "Cleanup any data and references, here.\n(this is called automatically, by the Macro: Exit)"
        n109 = Unbundle By Name(w280) -> ("Core.Current VI Reference"=w283:refnum<vi>)
        n110 = Close Reference(reference=w283, error in (no error)=w282) -> (error out=w281:errorcluster)
        n111 = call <vilib>:"Add State(s) to Queue__JKI_lib_State_Machine.vi"("State(s) in (\"\")"=w285) -> ("States Out"=w284:string)  [unwired: 14 in]
      }
      frame "---------- UI ----------" {
        # "Do not put any code in this frame.\n(It is a separator no-op. You can make a copy of this frame to create a new UI frame)"
        n112 = call <vilib>:"Add State(s) to Queue__JKI_lib_State_Machine.vi"("State(s) in (\"\")"=w290) -> ("States Out"=w289:string)  [unwired: 14 in]
      }
      frame "UI: Initialize" {
        n113 = control-ref of="Refresh Button"() -> (w295:refnum<vi>)
        n114 = control-ref of="Zoom Factor"() -> (w292:refnum<vi>)
        n115 = control-ref of="Splitter"() -> (w293:refnum<vi>)
        n116 = Build Array(w295, w292) -> (w294:refnum<vi>[])
        n117 = local write "Zoom Factor"(1.0 ("Zoom Factor")) -> ()
        n118 = call "Relocate Splitter Posistion.vi"("Array"=w294, "Splitter in"=w293) -> ()  [unwired: 9 in, 1 out]
        n119 = call <vilib>:"Add State(s) to Queue__JKI_lib_State_Machine.vi"("State(s) in (\"\")"=w300) -> ("States Out"=w299:string)  [unwired: 14 in]
      }
      frame "UI: Initialize Panel" {
        n120 = call <vilib>:"Set Busy.vi"() -> ("error out"=w305:errorcluster)  [unwired: 10 in, 1 out]
        n121 = call <vilib>:"Add State(s) to Queue__JKI_lib_State_Machine.vi"("State(s) in (\"\")"=w302, "State(s) at Back (\"\")"="UI: Clear Tree\nUI: Populate Ring\nUI: Group By Changed " ("State(s) at Back (\"\")")) -> ("States Out"=w303:string)  [unwired: 13 in]
      }
      frame "UI: Clear Tree" {
        n122 = invoke class="Tree (strict)" method="Edit Tree Items.Delete"(reference=refnum<vi> refnum, "Delete Children"=TRUE ("Delete Children?")) -> (reference out=w311:refnum<vi>, error out=w312:errorcluster)  [unwired: 3 in, 3 out]
        n123 = global read "User Visible Strings.vi" "Populating list"() -> (w313:string)
        n124 = invoke class="Tree (strict)" method="Edit Tree Items.Add Item"(reference=w311, error in=w312, "Left Cell"=w313) -> (reference out=w314:refnum<vi>, error out=w315:errorcluster)  [unwired: 6 in, 7 out]
        n125 = property class="Tree (strict)"(reference=w314, error in=w315, "DisabledEnum"=T8."Disabled" ("Disabled")) -> ()  [unwired: 2 out]
      }
      frame "UI: Group By Changed" {
        n126 = call <vilib>:"Add State(s) to Queue__JKI_lib_State_Machine.vi"("State(s) in (\"\")"=w320, "State(s) at Back (\"\")"="UI: Clear Tree\nUI: Start UI Update\nUI: Populate Tree\nUI: Finish UI Update" ("Message")) -> ("States Out"=w321:string)  [unwired: 13 in]
      }
      frame "UI: Start UI Update" {
        n127 = Unbundle By Name(w325) -> ("Front Panel"=w327:refnum<vi>)
        n128 = property class="Pnl"(reference=w327, "DeferPanUpdts"=TRUE ("Defer Panel Updates")) -> ()  [unwired: 1 in, 2 out]
        n129 = call <vilib>:"Set Busy.vi"() -> ()  [unwired: 10 in, 2 out]
      }
      frame "UI: Populate Tree" {
        n130 = Unbundle By Name(w332) -> ("App Info"=w335:T2)
        n131 = call "_Get Bookmarks.vi"("show vi in llb?"=FALSE, "App Info"=w335) -> ("error out"=w336:errorcluster, "bookmarks"=w334:T3[])  [unwired: 7 in, 1 out]
        n132 = Bundle By Name(cluster=w332, "bookmarks"=w334) -> (w333:T1)
      }
      frame "UI: Populate Ring" {
      }
      frame "UI: Populate Example Tree" {
        n133 = Unbundle By Name(w346) -> ("root"=w347:path)
        n134 = call "_List Example VIs.vi"("root"=w347) -> ("Array"=w351:path[])  [unwired: 10 in]
        n135 = Path To String(path=w351) -> (string=w342:string[])
        n136 = control-ref of="ExampleTree"() -> (w344:refnum<vi>)
        n137 = Build Array(w342) -> (w352:string[][])
        n138 = Transpose 2D Array(2D array=w352) -> (transposed array=w353:string[][])
        n139 = call "Populate Tree with Delimited Strings_csm.vi"("Use Child Only?"=TRUE, "Default Symbol"=26, "Delimiter"="\\", "Items (Delimited)"=w353, "Tree Control"=w344) -> ("error out"=w345:errorcluster)  [unwired: 4 in, 2 out]
      }
      frame "UI: Finish UI Update" {
        n140 = Unbundle By Name(w356) -> ("Front Panel"=w358:refnum<vi>)
        n141 = property class="Pnl"(reference=w358, "DeferPanUpdts"=FALSE ("Defer Panel Updates")) -> (error out=w355:errorcluster)  [unwired: 1 in, 1 out]
        n142 = call <vilib>:"Unset Busy.vi"("error in (no error)"=w355) -> ()  [unwired: 10 in, 1 out]
      }
      frame "UI: Highlight Bookmark" {
        n143 = call "CSM - Convert HexStr to Data.vi"("HEX String"=w363) -> ("Variant"=w364:variant, "error out"=w365:errorcluster)  [unwired: 7 in]
        n144 = Unbundle By Name(w367) -> ("bookmarks"=w372:T3[])
        n145 = Variant To Data(error in=w365, type="", Variant=w364) -> (data=w371:string, error out=w373:errorcluster)
        n146 = property class="Tree (strict)"(reference=refnum<vi> refnum, error in=w373, "Active Item Tag"=w371) -> (error out=w374:errorcluster, "Indent Level"=w369:i32)  [unwired: 1 out]
        n147 = Greater Than 0?(x=w369) -> (x > 0?=w370:bool)
        n148 = case shown="True" w370 {
          tunnel: w374 -> [w377 w383]
          tunnel: [w377 w380] -> w366
          tunnel: w371 -> [_ w382]
          tunnel: w372 -> [_ w381]
          frame False {
          }
          frame True {
            n149 = call "_Highlight Bookmark.vi"("error in (no error)"=w383, "bookmarks"=w381, "tag"=w382) -> ("error out"=w379:errorcluster)  [unwired: 8 in]
            n150 = call <vilib>:"Simple Error Handler.vi"("error in (no error)"=w379) -> ("error out"=w378:errorcluster)  [unwired: 4 in, 4 out]
            n151 = call <vilib>:"Clear Errors.vi"("error in (no error)"=w378) -> ("error out"=w380:errorcluster)  [unwired: 5 in, 1 out]
          }
        }
      }
      frame "UI: Highlight Doc" {
        w403 = FALSE ("Text.Font:Underline")
        n152 = local read "Doc"() -> (w396:string)
        n153 = control-ref of="BookmarkList"() -> (w422:refnum<vi>)
        n154 = property class="MCListbox (strict)"(reference=w422) -> ("ItemNames"=w420:string[][], "Value"=w421:i32)  [unwired: 1 in, 2 out]
        n155 = call "Text To Lines_CSM.vi"("Remove Empty Lines? (T)"=FALSE ("Remove Empty Lines?(T)"), "String"=w396) -> ("error out"=w416:errorcluster, "Lines"=w401:string[])  [unwired: 8 in]
        n156 = Index Array(array=w420, index (row)=w421) -> (element=w419:string[])  [unwired: 1 in]
        n157 = call "_Parse Markdown Doc Elements.vi"("Error in"=w416, "Lines"=w401) -> ("Error out"=w414:errorcluster, "Array"=w413:T9[], "Lines (dup)"=w415:string[])  [unwired: 7 in]
        n158 = Index Array(array=w419, index=0) -> (element=w410:string)
        n159 = call "_Parse Markdown Note Elements.vi"("Error in"=w414, "Lines"=w415) -> ("Array"=w412:T17[])  [unwired: 7 in, 2 out]
        n160 = Match Pattern(string=w410, regular expression="^#CSM-Example ") -> (after substring=w409:string)  [unwired: 1 in, 3 out]
        n161 = call "_Generate DocMap.vi"("Array 2"=w412, "Array"=w413) -> ("Variant"=w386:variant)  [unwired: 9 in]
        n162 = To Lower Case(string=w409) -> (all lower case string=w407:string)
        n163 = call "_Parse Markdown Steps.vi"("Variant"=w386) -> ("Variant 2"=w387:variant)  [unwired: 10 in]
        n164 = Get Variant Attribute(Variant=w387, name=w407, default value (empty Variant)=T9 {"ID"="", "Content"=[], "SubIDs"=[], "Path"=[]} ("output cluster")) -> (value=w406:T9)  [unwired: 1 in, 3 out]
        n165 = Unbundle By Name(w406) -> ("Content"=w405:string[])
        n166 = call "CSM - Compact Multiple States.vi"("Multiple States"=w405) -> ("States"=w404:string)  [unwired: 9 in]
        n167 = String Length(string=w404) -> (length=w402:i32)
        n168 = Search/Split String(string=w396, search string/char (-)=w404) -> (substring before match=w390:string, offset of match=w391:i32)  [unwired: 1 in, 1 out]
        n169 = Add(x=w391, y=w402) -> (x+y=w392:i32)
        n170 = control-ref of="Doc"() -> (w397:refnum<vi>)
        n171 = property class="Str"(reference=w397, "Text.Selection Start"=u32 0 ("Text.Selection:Start"), "Text.Selection End"=u32 4294967295 ("Text.Selection:Start"), "Text.FontColor"=u32 16777228) -> (reference out=w399:refnum<vi>, error out=w400:errorcluster)  [unwired: 1 in]
        n172 = call "CSM - Break Down Multiple States String.vi"("States"=w390) -> ("Multiple States"=w389:string[])  [unwired: 10 in]
        n173 = Array Size(array=w389) -> (size(s)=w385:i32)
        n174 = Subtract(x=w385, y=5) -> (x-y=w388:i32)
        n175 = property class="Str"(reference=w399, error in=w400, "Text.Selection Start"=w391, "Text.Selection End"=w392, "Text.FontColor"=u32 16711680, "Text.FontUnder"=w403, "Text.FontItalic"=w403, "Text.FontBold"=w403, "Text.Scroll Position"=w388) -> ()  [unwired: 2 out]
      }
      frame "UI: Change Image" {
        n176 = Unbundle By Name(w429) -> ()  [unwired: 1 out]
        n177 = call "CSM - Convert HexStr to Data.vi"("HEX String"=w430) -> ("Variant"=w427:variant, "error out"=w426:errorcluster)  [unwired: 7 in]
        n178 = Variant To Data(error in=w426, type="", Variant=w427) -> ()  [unwired: 2 out]
      }
      frame "UI: Change Image2" {
        n179 = control-ref of="BookmarkList"() -> (w443:refnum<vi>)
        n180 = property class="MCListbox (strict)"(reference=w443) -> ("ItemNames"=w441:string[][], "Value"=w442:i32)  [unwired: 1 in, 2 out]
        n181 = Unbundle By Name(w447) -> ("Preview image"=w446:refnum<vi>)
        n182 = Unbundle By Name(w437) -> ("tempfile"=w436:path)
        n183 = Index Array(array=w441, index (row)=w442) -> (element=w440:string[])  [unwired: 1 in]
        n184 = Index Array(array=w440, index=1) -> (element=w438:string)
        n185 = Decimal String To Number(string=w438) -> (number=w444:i32)  [unwired: 2 in, 1 out]
        n186 = call "_Change Bookmark Image.vi"("Picture Control Reference"=w446, "Bookmark ID"=w444, "vi path"=w436) -> ("error out"=w445:errorcluster)  [unwired: 8 in]
        n187 = call <vilib>:"Clear Errors.vi"("error in (no error)"=w445) -> ()  [unwired: 5 in, 2 out]
        n188 = call <vilib>:"Add State(s) to Queue__JKI_lib_State_Machine.vi"("State(s) in (\"\")"=w434, "State(s) at Back (\"\")"="UI: Change Zoom Factor" ("State(s) at Back (\"\")")) -> ("States Out"=w435:string)  [unwired: 13 in]
      }
      frame "UI: Change Doc" {
        n189 = disable-structure shown="Enabled" {
          disable-tunnel: [w457 w469] -> w450
          disable-tunnel: [w456 w466] -> w449
          disable-tunnel: w448 -> [w453 w469]
          frame Disabled {
            n190 = in-place {
              in-place-border: [w458] -> w454
              n191 = in-place-cluster #1(w453) -> ("DocMap"=w463:variant)
              n192 = local read "ExampleTree"() -> (w465:string)
              n193 = String To Path(string=w465) -> (path=w464:path)
              n194 = Strip Path(path=w464) -> (name=w461:string)  [unwired: 1 out]
              n195 = To Lower Case(string=w461) -> (all lower case string=w460:string)
              n196 = Get Variant Attribute(Variant=w463, name=w460, default value (empty Variant)=T9 {"ID"="", "Content"=[], "SubIDs"=[], "Path"=[]} ("Cluster")) -> (duplicate Variant=w462:variant, value=w458:T9)  [unwired: 1 in, 2 out]
              n197 = in-place-cluster #1("DocMap"=w462) -> (w457:T13)
            }
            n198 = Unbundle By Name(w454) -> ("Content"=w455:string[])
            n199 = call "CSM - Compact Multiple States.vi"("Multiple States"=w455) -> ("States"=w456:string)  [unwired: 9 in]
          }
          frame Enabled {
            n200 = Unbundle By Name(w469) -> ("tempfile"=w470:path)
            n201 = invoke class="App" method="Get VI.Description"("VI Path"=w470) -> ("VI Desc"=w467:string)  [unwired: 4 in, 4 out]
            n202 = call "CSM - Break Down Multiple States String.vi"("States"=w467) -> ("Multiple States"=w468:string[])  [unwired: 10 in]
            n203 = call "CSM - Compact Multiple States.vi"("Multiple States"=w468) -> ("States"=w466:string)  [unwired: 9 in]
          }
        }
        "Doc" <- w449
      }
      frame "UI: Cursor Set" {
        # "Argument"
        # "Set and Unset Cursor Busy.\n(Usage: \"UI: Cursor Set >> Busy|Idle\")"
        n204 = case shown="\"Idle\", Default" w472 {
          tunnel: w474 -> [w479 w481]
          tunnel: [w478 w480] -> w473
          frame "Idle", Default {
            n205 = call <vilib>:"Unset Busy.vi"("error in (no error)"=w479) -> ("error out"=w478:errorcluster)  [unwired: 10 in]
          }
          frame "Busy" {
            n206 = call <vilib>:"Set Busy.vi"("error in (no error)"=w481) -> ("error out"=w480:errorcluster)  [unwired: 9 in, 1 out]
          }
        }
        n207 = call <vilib>:"Add State(s) to Queue__JKI_lib_State_Machine.vi"("State(s) in (\"\")"=w477) -> ("States Out"=w476:string)  [unwired: 14 in]
      }
      frame "UI: Front Panel State" {
        # "Argument"
        # "Set Front Panel Open or Closed\n(Usage: \"UI: Front Panel State >> Open|Close\")"
        n208 = Unbundle By Name(w485) -> ("Core.Current VI Reference"=w484:refnum<vi>)
        n209 = case shown="\"Maximize\", \"Maximized\"" w483 {
          tunnel: w487 -> [w495 w510 w521 w534 w547]
          tunnel: [w497 w511 w523 w536 w549] -> w486
          tunnel: w484 -> [w496 w508 w522 w535 w548]
          frame "Open", "Standard", Default {
            w490 = T6."Standard" ("State")
            n210 = property class="VI"(reference=w496, error in=w495) -> (reference out=w493:refnum<vi>, error out=w494:errorcluster, "FP.State"=w492:T6)
            n211 = Not Equal?(x=w492, y=w490) -> (x != y?=w491:bool)
            n212 = case shown="True" w491 {
              tunnel: [w501 w503] -> w497
              tunnel: w494 -> [w500 w503]
              tunnel: w493 -> [w499 _]
              tunnel: w490 -> [w498 _]
              frame True {
                n213 = invoke class="VI" method="FP.Open"(reference=w499, error in=w500, "Activate"=TRUE, "State"=w498) -> (error out=w501:errorcluster)  [unwired: 1 in, 4 out]
              }
              frame False {
              }
            }
          }
          frame "Close", "Closed" {
            n214 = property class="VI"(reference=w508, error in=w510) -> (reference out=w507:refnum<vi>, error out=w509:errorcluster, "FP.State"=w505:T6)
            n215 = Not Equal?(x=w505, y=T6."Closed" ("Front Panel Window:State")) -> (x != y?=w504:bool)
            n216 = case shown="True" w504 {
              tunnel: [w512 w515] -> w511
              tunnel: w509 -> [w512 w514]
              tunnel: w507 -> [_ w513]
              frame False {
              }
              frame True {
                n217 = invoke class="VI" method="FP.Close"(reference=w513, error in=w514) -> (error out=w515:errorcluster)  [unwired: 1 in, 2 out]
              }
            }
          }
          frame "Hidden", "Hide" {
            w516 = T6."Hidden" ("State")
            n218 = property class="VI"(reference=w522, error in=w521) -> (reference out=w519:refnum<vi>, error out=w520:errorcluster, "FP.State"=w518:T6)
            n219 = Not Equal?(x=w518, y=w516) -> (x != y?=w517:bool)
            n220 = case shown="True" w517 {
              tunnel: [w527 w528] -> w523
              tunnel: w520 -> [w526 w528]
              tunnel: w519 -> [w525 _]
              tunnel: w516 -> [w524 _]
              frame True {
                n221 = invoke class="VI" method="FP.Open"(reference=w525, error in=w526, "State"=w524) -> (error out=w527:errorcluster)  [unwired: 2 in, 4 out]
              }
              frame False {
              }
            }
          }
          frame "Minimize", "Minimized" {
            w529 = T6."Minimized" ("State")
            n222 = property class="VI"(reference=w535, error in=w534) -> (reference out=w532:refnum<vi>, error out=w533:errorcluster, "FP.State"=w531:T6)
            n223 = Not Equal?(x=w531, y=w529) -> (x != y?=w530:bool)
            n224 = case shown="True" w530 {
              tunnel: [w540 w541] -> w536
              tunnel: w533 -> [w539 w541]
              tunnel: w532 -> [w538 _]
              tunnel: w529 -> [w537 _]
              frame True {
                n225 = invoke class="VI" method="FP.Open"(reference=w538, error in=w539, "State"=w537) -> (error out=w540:errorcluster)  [unwired: 2 in, 4 out]
              }
              frame False {
              }
            }
          }
          frame "Maximize", "Maximized" {
            w542 = T6."Maximized" ("State")
            n226 = property class="VI"(reference=w548, error in=w547) -> (reference out=w545:refnum<vi>, error out=w546:errorcluster, "FP.State"=w544:T6)
            n227 = Not Equal?(x=w544, y=w542) -> (x != y?=w543:bool)
            n228 = case shown="True" w543 {
              tunnel: [w553 w554] -> w549
              tunnel: w546 -> [w552 w554]
              tunnel: w545 -> [w551 _]
              tunnel: w542 -> [w550 _]
              frame True {
                n229 = invoke class="VI" method="FP.Open"(reference=w551, error in=w552, "State"=w550) -> (error out=w553:errorcluster)  [unwired: 2 in, 4 out]
              }
              frame False {
              }
            }
          }
        }
        n230 = call <vilib>:"Add State(s) to Queue__JKI_lib_State_Machine.vi"("State(s) in (\"\")"=w489) -> ("States Out"=w488:string)  [unwired: 14 in]
      }
      frame "UI: Change Zoom Factor" {
        n231 = case shown="Default" w556 {
          selector: w556 -> [_ w563]
          tunnel: [w562 w564] -> w557
          frame "" {
            n232 = local read "Zoom Factor"() -> (w562:dbl)
          }
          frame Default {
            n233 = Fract/Exp String To Number(string=w563) -> (number=w564:dbl)  [unwired: 3 in, 1 out]
          }
        }
        n234 = control-ref of="Preview"() -> (w555:refnum<vi>)
        n235 = property class="Pict"(reference=w555, "ZoomFactor"=w557) -> ()  [unwired: 1 in, 2 out]
      }
      frame "UI: Reset Bookmark List to Frist Row" {
        n236 = property on="BookmarkList" class="MCListbox (strict)"("TopLeft"=T10 {"Row"=0, "Column"=0} ("Top Left Visible Cell")) -> ()  [unwired: 2 in, 2 out]
      }
      frame "UI: Select First Example" {
        n237 = Unbundle By Name(w575) -> ("root"=w576:path)
        n238 = call "_List Example VIs.vi"("root"=w576) -> ("Array"=w577:path[])  [unwired: 10 in]
        n239 = Path To String(path=w577) -> (string=w574:string[])
        n240 = Index Array(array=w574) -> (element=w573:string)  [unwired: 1 in]
        n241 = property on="ExampleTree" class="Tree (strict)"("Val(Sgnl)"=w573) -> ()  [unwired: 2 in, 2 out]
        n242 = call <vilib>:"Add State(s) to Queue__JKI_lib_State_Machine.vi"("State(s) in Front (\"\")"="UI: Reset Bookmark List to Frist Row\nAction: Copy to tempfile\nAction: Refresh Example Description\nUI: Change Doc\nAction: Get Bookmarks\nUI: Change Image2" ("State(s) in Front (\"\")"), "State(s) in (\"\")"=w571) -> ("States Out"=w572:string)  [unwired: 13 in]
      }
      frame "---------- Macro ----------" {
        # "Do not put any code in this frame.\n(It is a separator no-op. You can make a copy of this frame to create a new Macro frame)"
        n243 = call <vilib>:"Add State(s) to Queue__JKI_lib_State_Machine.vi"("State(s) in (\"\")"=w584) -> ("States Out"=w583:string)  [unwired: 14 in]
      }
      frame "Macro: Initialize" {
        # "Initialization Macro\n(This is called once, when the VI starts)"
        n244 = call <vilib>:"Add State(s) to Queue__JKI_lib_State_Machine.vi"("State(s) in Front (\"\")"="Data: Initialize\nData: Initialize Refs\nInitialize Core Data\nUI: Initialize\nData: Search Example Markdowns\nData: Load Example Markdown Files\nUI: Populate Example Tree\nUI: Initialize Panel\nUI: Front Panel State >> Open\nUI: Select First Example\nMacro: Switch Example", "State(s) in (\"\")"=w590) -> ("States Out"=w589:string)  [unwired: 13 in]
      }
      frame "Macro: Switch Example" {
        n245 = call <vilib>:"Add State(s) to Queue__JKI_lib_State_Machine.vi"("State(s) in Front (\"\")"="Action: Copy to tempfile\nAction: Refresh Example Description\nUI: Change Doc\nAction: Get Bookmarks\nMacro: Switch Bookmark", "State(s) in (\"\")"=w596) -> ("States Out"=w595:string)  [unwired: 13 in]
      }
      frame "Macro: Switch Bookmark" {
        n246 = call <vilib>:"Add State(s) to Queue__JKI_lib_State_Machine.vi"("State(s) in Front (\"\")"="UI: Highlight Doc\nUI: Change Image2\nUI: Change Zoom Factor", "State(s) in (\"\")"=w602) -> ("States Out"=w601:string)  [unwired: 13 in]
      }
      frame "Macro: Exit" {
        # "Exit Macro\n(This is called once, when the VI exits)"
        n247 = Unbundle By Name(w610) -> ("Core.Close Panel on Exit?"=w609:bool)
        n248 = Select(t="UI: Front Panel State >> Close", s=w609, f="") -> (s? t:f=w606:string)
        n249 = call <vilib>:"Add State(s) to Queue__JKI_lib_State_Machine.vi"("State(s) in (\"\")"=w606, "State(s) at Back (\"\")"="Data: Cleanup\nExit") -> ("States Out"=w604:string)  [unwired: 13 in]
        n250 = call <vilib>:"Add State(s) to Queue__JKI_lib_State_Machine.vi"("State(s) in Front (\"\")"=w604, "State(s) in (\"\")"=w613) -> ("States Out"=w612:string)  [unwired: 13 in]
      }
      frame "---------- New Category ----------" {
        # "Template Separator\n(You can make a copy of, or modify, this frame)"
        n251 = call <vilib>:"Add State(s) to Queue__JKI_lib_State_Machine.vi"("State(s) in (\"\")"=w618) -> ("States Out"=w617:string)  [unwired: 14 in]
      }
      frame "Action: Get Bookmarks" {
        n252 = local read "ExampleTree"() -> (w621:string)
        n253 = Unbundle By Name(w620) -> ("root"=w624:path)
        n254 = Unbundle By Name(w620) -> ("tempfile"=w619:path)
        n255 = Build Path(base path=w624, name or relative path=w621) -> ()  [unwired: 1 out]
        n256 = invoke class="App" method="Get VI.Bookmarks"("VIPath"=w619) -> ("BookmarkInfo"=w623:T18)  [unwired: 4 in, 4 out]
        n257 = call "_BMarkInfo to MCTable.vi"("BookmarkInfo"=w623) -> ("sorted 2D array"=w622:string[][])  [unwired: 10 in]
        n258 = property on="BookmarkList" class="MCListbox (strict)"("ItemNames"=w622) -> ()  [unwired: 2 in, 2 out]
      }
      frame "Action: Refresh Example Description" {
        n259 = disable-structure shown="Enabled" {
          disable-tunnel: w629 -> [w633 w652]
          disable-tunnel: [w632 w652] -> w628
          frame Disabled {
            n260 = in-place {
              n261 = in-place-cluster #2(w633) -> ("tempfile"=w634:path, "root"=w635:path, "DocMap"=w649:variant)
              n262 = local read "ExampleTree"() -> (w651:string)
              n263 = String To Path(string=w651) -> (path=w650:path)
              n264 = Strip Path(path=w650) -> (name=w647:string)  [unwired: 1 out]
              n265 = To Lower Case(string=w647) -> (all lower case string=w646:string)
              n266 = Get Variant Attribute(Variant=w649, name=w646, default value (empty Variant)=T9 {"ID"="", "Content"=[], "SubIDs"=[], "Path"=[]} ("Cluster")) -> (duplicate Variant=w648:variant, value=w644:T9)  [unwired: 1 in, 2 out]
              n267 = Unbundle By Name(w644) -> ("Content"=w643:string[])
              n268 = call "1D Array to String_csm.vi"("delimiter (Tab)"="\r", "Array of Strings"=w643) -> ("delimited string"=w639:string)  [unwired: 9 in]
              n269 = call <vilib>:"Trim Whitespace.vi"("string"=w639) -> ("trimmed string"=w638:string)  [unwired: 1 in]
              n270 = call "Populate Single Example Description.vi"("Show FP"=FALSE, "VI Description"=w638, "Path"=w634) -> ("error out"=w641:errorcluster)  [unwired: 8 in]
              n271 = call "Stall Data Flow.vim"("value in"=w641, "milliseconds to wait"=u32 100) -> ("value out"=w637:errorcluster)  [unwired: 1 out]
              n272 = in-place-cluster #2("tempfile"=w634, "root"=w635, "DocMap"=w648) -> (w632:T13)
              n273 = call <vilib>:"Clear Errors.vi"("error in (no error)"=w637) -> ()  [unwired: 5 in, 2 out]
            }
          }
          frame Enabled {
          }
        }
      }
      frame "Action: Copy to tempfile" {
        n274 = local read "ExampleTree"() -> (w658:string)
        n275 = Unbundle By Name(w657) -> ("root"=w659:path)
        n276 = Build Path(base path=w659, name or relative path=w658) -> (appended path=w656:path)
        n277 = disable-structure shown="Enabled" {
          disable-tunnel: w656 -> [w670 w671]
          disable-tunnel: [w664 w671] -> w654
          disable-tunnel: [w663 _] -> w653
          frame Disabled {
            n278 = call "uuid.vi"() -> ("UUID"=w668:string)  [unwired: 11 in]
            n279 = Temporary Directory() -> (w665:path)
            n280 = Concatenate Strings(w668, ".vi" ("string")) -> (w666:string)
            n281 = Build Path(base path=w665, name or relative path=w666) -> (appended path=w664:path)
            n282 = Copy(9:TRUE ("overwrite (F)"), 10:w664, 11:w670) -> (0:w663:errorcluster)  [unwired: 2 in, 2 out]
          }
          frame Enabled {
          }
        }
        n283 = Bundle By Name(cluster=w657, "tempfile"=w654) -> (w655:T13)
        n284 = call <vilib>:"Add State(s) to Queue__JKI_lib_State_Machine.vi"("State(s) in (\"\")"=w662) -> ("States Out"=w661:string)  [unwired: 14 in]
      }
      frame "Menu: PREVIEW_OPEN_VI" {
        n285 = local read "ExampleTree"() -> (w676:string)
        n286 = Unbundle By Name(w675) -> ("root"=w677:path)
        n287 = Build Path(base path=w677, name or relative path=w676) -> (appended path=w674:path)
        n288 = call <vilib>:"Check if File or Folder Exists.vi"("path"=w674) -> ("file or folder exists?"=w672:bool, "dup path"=w673:path)  [unwired: 8 in, 1 out]
        n289 = case shown="True" w672 {
          tunnel: w673 -> [_ w683]
          frame False {
          }
          frame True {
            n290 = Open VI Reference(vi path=w683, options=2) -> (vi reference=w686:refnum<vi>, error out=w688:errorcluster)  [unwired: 4 in]
            n291 = property class="VI"(reference=w686, error in=w688, "BDWin.Open"=TRUE ("Block Diagram Window:Open")) -> (reference out=w684:refnum<vi>, error out=w685:errorcluster)
            n292 = Close Reference(reference=w684, error in (no error)=w685) -> ()  [unwired: 1 out]
          }
        }
        n293 = call <vilib>:"Add State(s) to Queue__JKI_lib_State_Machine.vi"("State(s) in (\"\")"=w681) -> ("States Out"=w680:string)  [unwired: 14 in]
      }
    }
  }
  n294 = control-ref of="Current VI Reference"() -> (w2:refnum<vi>)
  n295 = call "Close FP if in LabVIEW Dir.vi"("VI Refnum"=w2, "Error in"=w1) -> ("Error out"=w3:errorcluster)  [unwired: 9 in]
  n296 = call <vilib>:"Clear Errors.vi"("error in (no error)"=w3) -> ()  [unwired: 5 in, 2 out]
